vi "ER2007 Calibration Panel.vi"() -> ()   [LabVIEW 2013]
doc: "This vi is used to display and assign calibration parameters to A/D, D/A, and digital I/O channels. These parameters are grouped by channel type (i.e., A/D, D/A, etc) and displayed on separate pages. The user selects a page for review and/or modification using the text ring at the top of the page; changes to a page are saved by pressing the \"Save Page\" button. The calibration coefficients are used to convert voltages to engineering values and vice versa. When a channel is re-calibrated, the new coefficients should be entered here. To permanently store changes, you must press \"Save Page\" for the appropriate channel first. This enables the \"OK\" button at the bottom right of the screen; press this button to save the new value(s) to the calibration file. (The calibration file is read at startup inside the Main Panel vi.) Press \"Cancel\" to restore previous values. AutoCon, Inc., 6/98"
uses:
  Controls/Global ER2007.vi
panel:
  in  "Set":bool
  out "VersionLabel":string="Program JackScrew, Version 0.01, Rolls Royce Gear Systems, Copyright 2000, All Rights Reserved"
  in  "OK":bool
  in  "Cancel":bool
  in  "SavePage":bool
  in  "HW Configuration":u16[](array[ring]) items=["Not Configured", "Bipolar, -10V to +10V", "Unipolar, 0 to +10V", "Bipolar, -5V to +5V", "Unipolar, 0 to +5V", "<reserved>", "<reserved>", "<reserved>", "<reserved>", "<reserved>", "<reserved>", "Digital Input", "Digital Output", "Counter Input"]
  in  "Factor":sgl[](array[numeric]) format="%.5f"
  in  "Zeroes":sgl[](array[numeric]) format="%.5f"
  in  "Page #":u16(ring) items=["Dev 1 PCI-6220 Port 0 DigOut Chls 0-7 DOUT", "Dev 1 PCI-6220 Port 1 DigOut Chls 0-7 DOUT", "Dev 1 PCI-6220 Port 2 DigIn Chls 0-7 DIN", "Dev 1 PCI-6220 Analog In Chls 0-15 AIN", "Dev 2 PCI-6224 Port 0 DigOut Chls 0-7 DOUT", "Dev 2 PCI-6224 Port 0 DigOut Chls 8-15 DOUT", "Dev 2 PCI-6224 Port 1 DigOut Chls 0-7 DOUT", "Dev 2 PCI-6224 Port 2 DigIn Chls 0-7 DIN", "Dev 2 PCI-6224 Analog In Chls 0-15 AIN", "Dev 2 PCI-6224 Analog In Chls 16-31 AIN", "Net 0 Galil CDS 3310", "GPIB 0 IEEE-488 Interface Addr"]
  out "Chl #":string[](array[string])
  in  "Channel Description":string[](array[string])
  in  "Units":string[](array[string])
  # "Calibration Panel"
  # "Note: Units of \"psia\", \"Volts\" and\n\"deg-C\" have special zero routines"
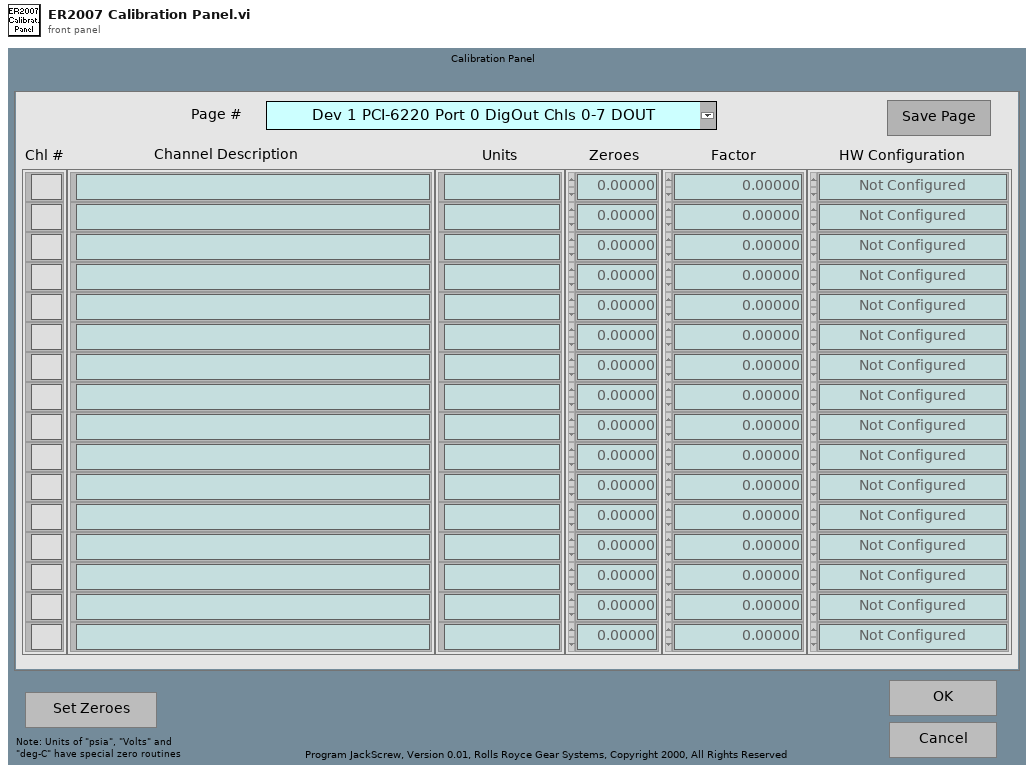
[diagram p1: front panel]
types:
  T1 = cluster{"PageTitle":string, "NumLines":i32, "ChlNum":string[], "ChlDesc":string[], "ChlUnits":string[], "ChlZero":sgl[], "ChlFactor":sgl[], "ChlConfig":u16[]}[]
  T2 = cluster{"PageTitle":string, "NumLines":i32, "ChlNum":string[], "ChlDesc":string[], "ChlUnits":string[], "ChlZero":sgl[], "ChlFactor":sgl[], "ChlConfig":u16[]}
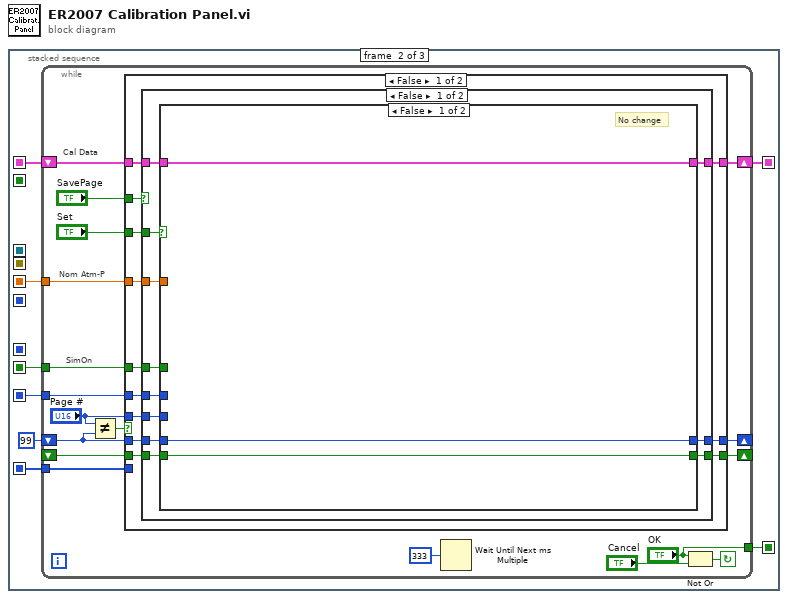
[diagram p0: block diagram]
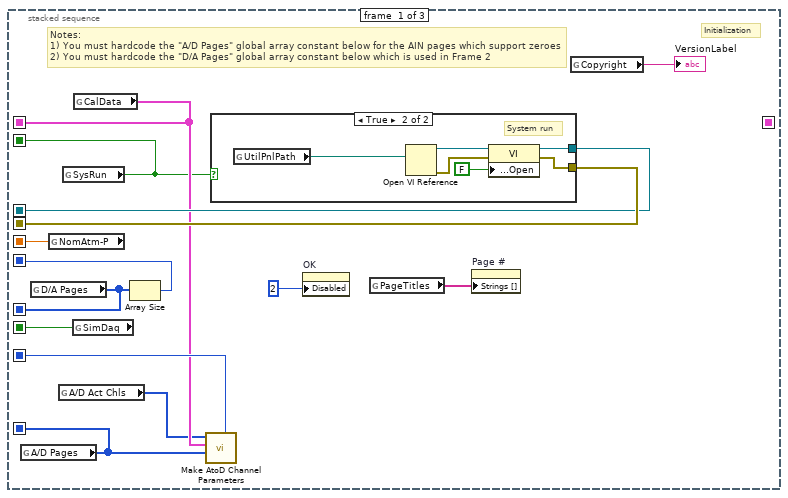
[diagram p2: hidden frame]
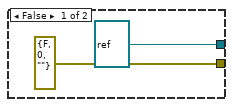
[diagram p3: hidden frame]
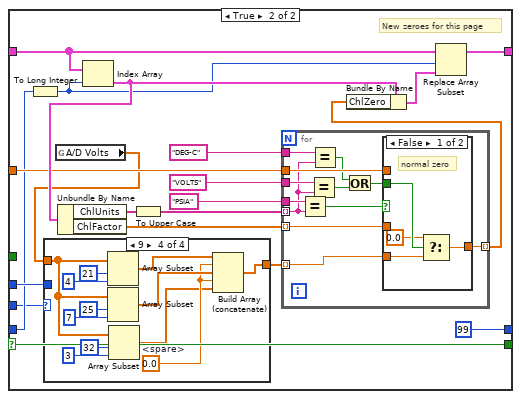
[diagram p5: hidden frame]
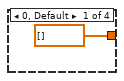
[diagram p6: hidden frame]
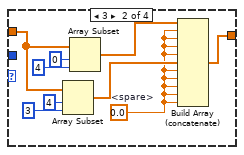
[diagram p7: hidden frame]
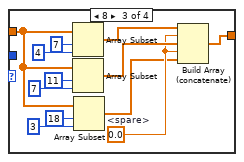
[diagram p8: hidden frame]
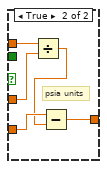
[diagram p9: hidden frame]
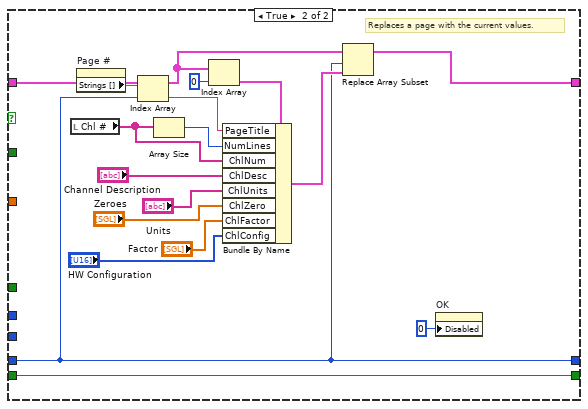
[diagram p10: hidden frame]
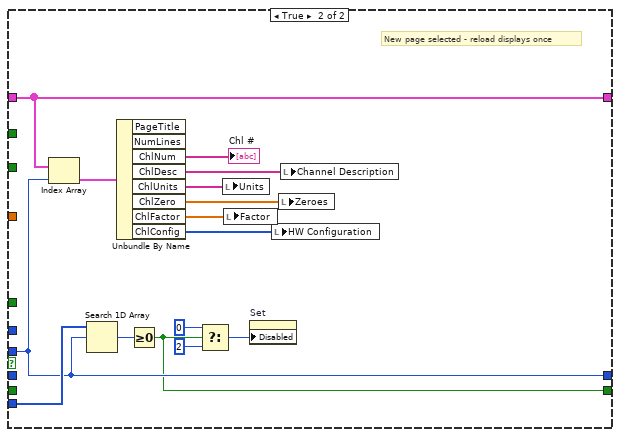
[diagram p11: hidden frame]
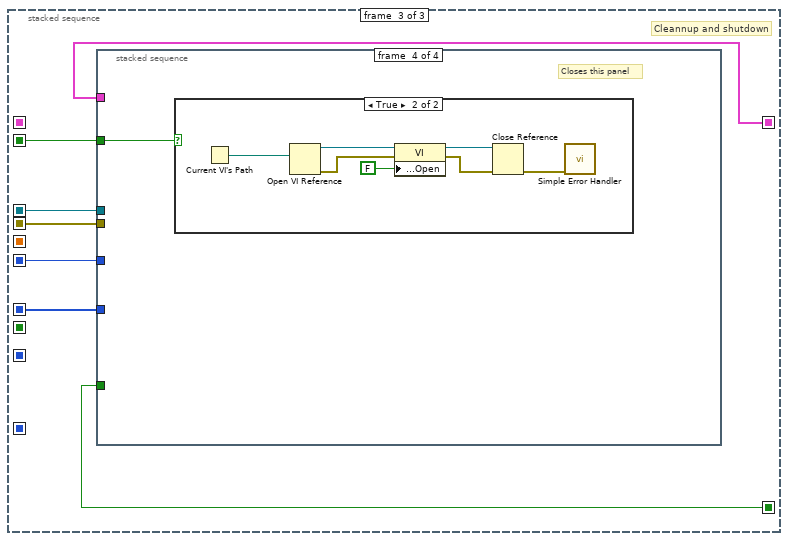
[diagram p12: hidden frame]
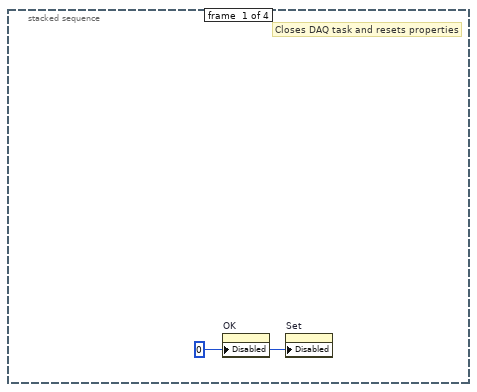
[diagram p13: hidden frame]
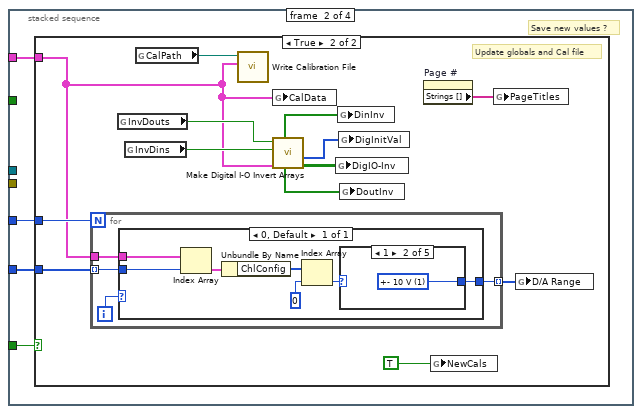
[diagram p14: hidden frame]
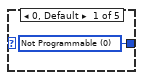
[diagram p16: hidden frame]
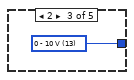
[diagram p17: hidden frame]
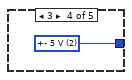
[diagram p18: hidden frame]
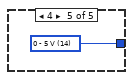
[diagram p19: hidden frame]
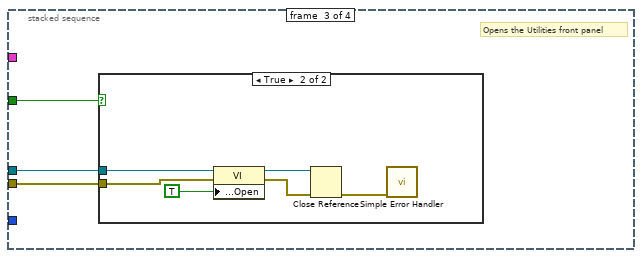
[diagram p20: hidden frame]
diagram:
  n1 = stacked-sequence {
    seq-local: [_ w28 _] -> [_ _ w201]
    seq-local: [w8 _ _] -> [_ w30 _]
    seq-local: [_ w27 _] -> [_ _ w200]
    seq-local: [w4 _ _] -> [_ w26 _]
    seq-local: [w6 _ _] -> [_ w25 _]
    seq-local: [w2 _ _] -> [_ w24 _]
    seq-local: [w13 _ _] -> [_ _ w199]
    seq-local: [w5 _ _] -> [_ _ w198]
    seq-local: [w12 _ _] -> [_ w23 _]
    seq-local: [w7 _ _] -> [_ _ w197]
    seq-local: [w10 _ _] -> [_ _ w196]
    seq-local: [w11 _ _] -> [_ _ w195]
    frame #0 {
      # "Notes:\n1) You must hardcode the \"A/D Pages\" global array constant below for the AIN pages which support zeroes\n2) You must hardcode the \"D/A Pages\" global array constant below which is used in Frame 2"
      # "Initialization"
      n2 = global read "Global ER2007.vi" "A/D Pages"() -> (w2:i32[])
      n3 = global read "Global ER2007.vi" "D/A Pages"() -> (w5:i32[])
      n4 = global read "Global ER2007.vi" "NomAtm-P"() -> (w6:dbl)
      n5 = global read "Global ER2007.vi" "A/D Act Chls"() -> (w3:i32[])
      n6 = global read "Global ER2007.vi" "SysRun"() -> (w7:bool)
      n7 = global read "Global ER2007.vi" "SimDaq"() -> (w4:bool)
      n8 = global read "Global ER2007.vi" "CalData"() -> (w8:T1)
      n9 = Array Size(array=w5) -> (size(s)=w13:i32)
      n10 = call "Make AtoD Channel Parameters.vi"("A/D Pages"=w2, "CalData"=w8, "A/D Active Chl List"=w3) -> ("NumChls"=w12:i32)  [unwired: 2 in, 6 out]
      n11 = case shown="True" w7 {
        tunnel: [refnum<vi> refnum w19] -> w10
        tunnel: [errorcluster {"status"=FALSE, "code"=0, "source"=""} ("error out") w18] -> w11
        frame False {
        }
        frame True {
          # "System run"
          n12 = global read "Global ER2007.vi" "UtilPnlPath"() -> (w17:path)
          n13 = Open VI Reference(vi path=w17) -> (vi reference=w22:refnum<vi>, error out=w21:errorcluster)  [unwired: 5 in]
          n14 = property class="VI"(reference=w22, error in=w21, "Front Panel Window:Open"=FALSE) -> (reference out=w19:refnum<vi>, error out=w18:errorcluster)
        }
      }
      n15 = property on="OK" class="Bool"("Disabled"=u8 2) -> ()  [unwired: 2 in, 2 out]
      n16 = global read "Global ER2007.vi" "PageTitles"() -> (w1:string[])
      n17 = property on="Page #" class="Ring (strict)"("Strings []"=w1) -> ()  [unwired: 2 in, 2 out]
      n18 = global read "Global ER2007.vi" "Copyright"() -> (→"VersionLabel":string)
    }
    frame #1 {
      n19 = while {
        tunnel: w25 -> [w35]
        tunnel: w26 -> [w36]
        tunnel: ["OK"] -> w28
        shift-left: u16 99 -> [w46]
        shift-right: [w44] -> _
        shift-left: w30 -> [w47]
        shift-right: [w43] -> w27
        tunnel: w24 -> [w34]
        tunnel: w23 -> [w33]
        shift-right: [w32] -> _
        shift-left: _ -> [w31]
        stop <- w40 continue-if-true
        # "Cal Data"
        # "SimOn"
        # "Nom Atm-P"
        n20 = Not Equal?(x="Page #", y=w46) -> (x != y?=w48:bool)
        n21 = case shown="False" w48 {
          tunnel: w47 -> [w60 w194]
          tunnel: w46 -> [w57 _]
          tunnel: "Page #" -> [w49 w183]
          tunnel: [w56 w183] -> w44
          tunnel: [w59 w194] -> w43
          tunnel: "SavePage" -> [w58 _]
          tunnel: "Set" -> [w55 _]
          tunnel: w36 -> [w54 _]
          tunnel: w35 -> [w53 _]
          tunnel: w34 -> [_ w184]
          tunnel: w33 -> [w52 _]
          tunnel: [w50 w181] -> w32
          tunnel: w31 -> [w51 _]
          frame False {
            n22 = case shown="False" w58 {
              tunnel: w60 -> [w70 w171]
              tunnel: [w71 w169] -> w59
              tunnel: w57 -> [w67 w165]
              tunnel: [w68 w165] -> w56
              tunnel: w55 -> [w69 _]
              tunnel: w54 -> [w66 _]
              tunnel: w53 -> [w65 _]
              tunnel: w52 -> [w64 _]
              tunnel: w51 -> [w63 w164]
              tunnel: [w62 w164] -> w50
              tunnel: w49 -> [w61 _]
              frame False {
                n23 = case shown="False" w69 {
                  tunnel: [w74 w83] -> w71
                  tunnel: w70 -> [w74 w82]
                  tunnel: [w73 w84] -> w68
                  tunnel: w67 -> [w73 w77]
                  tunnel: w66 -> [_ w81]
                  tunnel: w65 -> [_ w80]
                  tunnel: w64 -> [_ w79]
                  tunnel: w63 -> [w72 w78]
                  tunnel: [w72 w76] -> w62
                  tunnel: w61 -> [_ w75]
                  frame False {
                    # "No change"
                  }
                  frame True {
                    n24 = case shown="False" w78 {
                      selector: w78 -> [w86 w92]
                      tunnel: [w85 u16 99] -> w84
                      tunnel: [w87 w104] -> w83
                      tunnel: w82 -> [w87 w103]
                      tunnel: w81 -> [_ _]
                      tunnel: w80 -> [_ w96]
                      tunnel: w79 -> [_ w93]
                      tunnel: w77 -> [w85 w90]
                      tunnel: [w86 w92] -> w76
                      tunnel: w75 -> [_ w89]
                      frame False {
                        # "This page does not support zeroing"
                      }
                      frame True {
                        # "New zeroes for this page"
                        n25 = To Long Integer(number=w90) -> (32bit integer=w100:i32)
                        n26 = global read "Global ER2007.vi" "A/D Volts"() -> (w88:dbl[])
                        n27 = case shown="9" w89 {
                          tunnel: [dbl[] [] w114 w118 w130] -> w95
                          tunnel: w93 -> [_ _ _ _]
                          tunnel: w88 -> [_ w111 w120 w132]
                          frame 0, Default {
                          }
                          frame 3 {
                            w109 = 0.0  # <spare>
                            n28 = Array Subset(array=w111, index=4, length=3) -> (w110:dbl[])
                            n29 = Array Subset(array=w111, index=0, length=4) -> (w115:dbl[])
                            n30 = Build Array (concatenate)(w115, w109, w109, w109, w109, w110, w109, w109, w109, w109, w109) -> (w114:dbl[])
                          }
                          frame 8 {
                            w121 = 0.0  # <spare>
                            n31 = Array Subset(array=w120, index=7, length=4) -> (w127:dbl[])
                            n32 = Array Subset(array=w120, index=11, length=7) -> (w124:dbl[])
                            n33 = Array Subset(array=w120, index=18, length=3) -> (w119:dbl[])
                            n34 = Build Array (concatenate)(w127, w121, w124, w121, w119) -> (w118:dbl[])
                          }
                          frame 9 {
                            w133 = 0.0  # <spare>
                            n35 = Array Subset(array=w132, index=21, length=4) -> (w139:dbl[])
                            n36 = Array Subset(array=w132, index=25, length=7) -> (w136:dbl[])
                            n37 = Array Subset(array=w132, index=32, length=3) -> (w131:dbl[])
                            n38 = Build Array (concatenate)(w139, w133, w136, w133, w131) -> (w130:dbl[])
                          }
                        }
                        n39 = Index Array(array=w103, index=w100) -> (element=w102:T2)
                        n40 = Unbundle By Name(w102) -> ("ChlUnits"=w107:string[], "ChlFactor"=w99:sgl[])
                        n41 = To Upper Case(1:w107) -> (0:w106:string[])
                        n42 = for {
                          tunnel: w95 -> [w142] mode=indexing
                          tunnel: w106 -> [w147] mode=indexing
                          tunnel: "PSIA" -> [w153]
                          tunnel: [w151] -> w98 mode=indexing
                          tunnel: w99 -> [w150] mode=indexing
                          tunnel: w96 -> [w149]
                          tunnel: "VOLTS" -> [w148]
                          tunnel: "DEG-C" -> [w146]
                          n43 = Equal?(x=w153, y=w147) -> (x = y?=w152:bool)
                          n44 = Equal?(x=w148, y=w147) -> (x = y?=w144:bool)
                          n45 = Equal?(x=w146, y=w147) -> (x = y?=w143:bool)
                          n46 = Or(x=w143, y=w144) -> (x .or. y?=w145:bool)
                          n47 = case shown="False" w152 {
                            tunnel: [w154 w159] -> w151
                            tunnel: w142 -> [w156 w160]
                            tunnel: w150 -> [_ w161]
                            tunnel: w149 -> [_ w162]
                            tunnel: w145 -> [w157 _]
                            frame False {
                              # "normal zero"
                              n48 = Select(t=0.0, s=w157, f=w156) -> (s? t:f=w154:dbl)
                            }
                            frame True {
                              # "psia units"
                              n49 = Divide(x=w162, y=w161) -> (x/y=w158:dbl)
                              n50 = Subtract(x=w160, y=w158) -> (x-y=w159:dbl)
                            }
                          }
                        }
                        n51 = Bundle By Name(cluster=w102, "ChlZero"=w98) -> (w101:T2)
                        n52 = Replace Array Subset(array=w103, new element=w101, index=w100) -> (w104:T1)
                      }
                    }
                  }
                }
              }
              frame True {
                # "Replaces a page with the current values."
                n53 = local read "Chl #"() -> (w163:string[])
                n54 = property on="Page #" class="Ring (strict)"() -> ("Strings []"=w168:string[])  [unwired: 2 in, 2 out]
                n55 = Index Array(array=w168, index=w165) -> (element=w167:string)
                n56 = Array Size(array=w163) -> (size(s)=w172:i32)
                n57 = Index Array(array=w171, index=0 ("Index")) -> (element=w178:T2)
                n58 = Bundle By Name(cluster=w178, "PageTitle"=w167, "NumLines"=w172, "ChlNum"=w163, "ChlDesc"="Channel Description", "ChlUnits"="Units", "ChlZero"="Zeroes", "ChlFactor"="Factor", "ChlConfig"="HW Configuration") -> (w170:T2)
                n59 = Replace Array Subset(array=w171, new element=w170, index=w165) -> (w169:T1)
                n60 = property on="OK" class="Bool"("Disabled"=u8 0) -> ()  [unwired: 2 in, 2 out]
              }
            }
          }
          frame True {
            # "New page selected - reload displays once"
            n61 = Index Array(array=w194, index=w183) -> (element=w193:T2)
            n62 = Search 1D Array(1D array=w184, element=w183) -> (index of element=w182:i32)  [unwired: 1 in]
            n63 = Unbundle By Name(w193) -> ("ChlNum"=→"Chl #":string[], "ChlDesc"=w188:string[], "ChlUnits"=w189:string[], "ChlZero"=w190:sgl[], "ChlFactor"=w191:sgl[], "ChlConfig"=w192:u16[])  [unwired: 2 out]
            n64 = Greater Or Equal To 0?(x=w182) -> (x >= 0?=w181:bool)
            n65 = Select(t=u8 0 ("Disabled"), s=w181, f=u8 2) -> (s? t:f=w186:u8)
            n66 = local write "Units"(w189) -> ()
            n67 = local write "Factor"(w191) -> ()
            n68 = property on="Set" class="Bool"("Disabled"=w186) -> ()  [unwired: 2 in, 2 out]
            n69 = local write "HW Configuration"(w192) -> ()
            n70 = local write "Zeroes"(w190) -> ()
            n71 = local write "Channel Description"(w188) -> ()
          }
        }
        n72 = Wait Until Next ms Multiple(millisecond multiple=u32 333) -> ()  [unwired: 1 out]
        n73 = Not Or(1:"Cancel", 2:"OK") -> (0:w40:bool)
      }
    }
    frame #2 {
      # "Cleannup and shutdown"
      n74 = stacked-sequence {
        tunnel: w201 -> [_ w206 _ _]
        tunnel: w200 -> [_ w205 _ _]
        tunnel: w199 -> [_ w204 _ _]
        tunnel: w198 -> [_ w203 _ _]
        tunnel: w197 -> [_ _ w238 w245]
        tunnel: w196 -> [_ _ w237 _]
        tunnel: w195 -> [_ _ w236 _]
        frame #0 {
          w202 = u8 0 ("Write Attribute")
          # "Closes DAQ task and resets properties"
          n75 = property on="OK" class="Bool"("Disabled"=w202) -> ()  [unwired: 2 in, 2 out]
          n76 = property on="Set" class="Bool"("Disabled"=w202) -> ()  [unwired: 2 in, 2 out]
        }
        frame #1 {
          # "Save new values ?"
          n77 = case shown="True" w206 {
            tunnel: w205 -> [_ w208]
            tunnel: w204 -> [_ w219]
            tunnel: w203 -> [_ w218]
            frame False {
            }
            frame True {
              # "Update globals and Cal file"
              n78 = for {
                N: w219 -> [_]
                tunnel: w208 -> [w222]
                tunnel: [w221] -> w209 mode=indexing
                tunnel: w218 -> [w220] mode=indexing
                i -> [w223]
                n79 = case shown="0, Default" w223 {
                  tunnel: w222 -> [w225]
                  tunnel: [w226] -> w221
                  tunnel: w220 -> [w224]
                  frame 0, Default {
                    n80 = Index Array(array=w225, index=w224) -> (element=w230:T2)
                    n81 = Unbundle By Name(w230) -> ("ChlConfig"=w229:u16[])
                    n82 = Index Array(array=w229, index=0 ("Index")) -> (element=w227:u16)
                    n83 = case shown="1" w227 {
                      tunnel: [w231 w232 w233 w234 w235] -> w226
                      frame 0, Default {
                        w231 = 0 items=["Not Programmable", "+- 10 V", "+- 5 V", "+- 2.5 V", "+- 1.67 V", "+- 1.25 V", "+- 1 V", "+- .625 V", "+- .5 V", "+- .1 V", "+- .05 V", "+- .01 V", "+- .005 V", "0 - 10 V", "0 - 5 V", "0 - 2.5 V", "0 - 2 V", "0 - 1.67 V", "0 - 1.25 V", "0 - 1 V", "0 - .1 V", "0 - .01 V", "4-20 mA", "2-10 mA", "1-5 mA", "0.5-2.5 mA"] ("DA0Range")
                      }
                      frame 1 {
                        w232 = 1 items=["Not Programmable", "+- 10 V", "+- 5 V", "+- 2.5 V", "+- 1.67 V", "+- 1.25 V", "+- 1 V", "+- .625 V", "+- .5 V", "+- .1 V", "+- .05 V", "+- .01 V", "+- .005 V", "0 - 10 V", "0 - 5 V", "0 - 2.5 V", "0 - 2 V", "0 - 1.67 V", "0 - 1.25 V", "0 - 1 V", "0 - .1 V", "0 - .01 V", "4-20 mA", "2-10 mA", "1-5 mA", "0.5-2.5 mA"] ("DA0Range")
                      }
                      frame 2 {
                        w233 = 13 items=["Not Programmable", "+- 10 V", "+- 5 V", "+- 2.5 V", "+- 1.67 V", "+- 1.25 V", "+- 1 V", "+- .625 V", "+- .5 V", "+- .1 V", "+- .05 V", "+- .01 V", "+- .005 V", "0 - 10 V", "0 - 5 V", "0 - 2.5 V", "0 - 2 V", "0 - 1.67 V", "0 - 1.25 V", "0 - 1 V", "0 - .1 V", "0 - .01 V", "4-20 mA", "2-10 mA", "1-5 mA", "0.5-2.5 mA"] ("DA0Range")
                      }
                      frame 3 {
                        w234 = 2 items=["Not Programmable", "+- 10 V", "+- 5 V", "+- 2.5 V", "+- 1.67 V", "+- 1.25 V", "+- 1 V", "+- .625 V", "+- .5 V", "+- .1 V", "+- .05 V", "+- .01 V", "+- .005 V", "0 - 10 V", "0 - 5 V", "0 - 2.5 V", "0 - 2 V", "0 - 1.67 V", "0 - 1.25 V", "0 - 1 V", "0 - .1 V", "0 - .01 V", "4-20 mA", "2-10 mA", "1-5 mA", "0.5-2.5 mA"] ("DA0Range")
                      }
                      frame 4 {
                        w235 = 14 items=["Not Programmable", "+- 10 V", "+- 5 V", "+- 2.5 V", "+- 1.67 V", "+- 1.25 V", "+- 1 V", "+- .625 V", "+- .5 V", "+- .1 V", "+- .05 V", "+- .01 V", "+- .005 V", "0 - 10 V", "0 - 5 V", "0 - 2.5 V", "0 - 2 V", "0 - 1.67 V", "0 - 1.25 V", "0 - 1 V", "0 - .1 V", "0 - .01 V", "4-20 mA", "2-10 mA", "1-5 mA", "0.5-2.5 mA"] ("DA0Range")
                      }
                    }
                  }
                }
              }
              n84 = global read "Global ER2007.vi" "InvDouts"() -> (w216:bool)
              n85 = global read "Global ER2007.vi" "InvDins"() -> (w215:bool)
              n86 = global read "Global ER2007.vi" "CalPath"() -> (w217:path)
              n87 = call "Write Calibration File.vi"("CalDataIn"=w208, "CalFilepath"=w217) -> ()  [unwired: 6 in]
              n88 = global write "Global ER2007.vi" "CalData"(w208) -> ()
              n89 = call "Make Digital I-O Invert Arrays.vi"("CalDataIn"=w208, "InvDins"=w215, "InvDouts"=w216) -> ("DIO-Inv"=w212:bool[][], "DoutInit"=w211:i32[], "DoutInv (1D)"=w213:bool[], "DinInv (1D)"=w214:bool[])  [unwired: 1 in, 4 out]
              n90 = global write "Global ER2007.vi" "DigIO-Inv"(w212) -> ()
              n91 = global write "Global ER2007.vi" "DinInv"(w214) -> ()
              n92 = global write "Global ER2007.vi" "DigInitVal"(w211) -> ()
              n93 = global write "Global ER2007.vi" "DoutInv"(w213) -> ()
              n94 = property on="Page #" class="Ring (strict)"() -> ("Strings []"=w210:string[])  [unwired: 2 in, 2 out]
              n95 = global write "Global ER2007.vi" "NewCals"(TRUE ("NewCals")) -> ()
              n96 = global write "Global ER2007.vi" "PageTitles"(w210) -> ()
              n97 = global write "Global ER2007.vi" "D/A Range"(w209) -> ()
            }
          }
        }
        frame #2 {
          # "Opens the Utilities front panel"
          n98 = case shown="True" w238 {
            tunnel: w237 -> [_ w244]
            tunnel: w236 -> [_ w243]
            frame False {
              # "Not a System run"
            }
            frame True {
              n99 = property class="VI"(reference=w244, error in=w243, "Front Panel Window:Open"=TRUE) -> (reference out=w241:refnum<vi>, error out=w240:errorcluster)
              n100 = Close Reference(reference=w241, error in (no error)=w240) -> (error out=w239:errorcluster)
              n101 = call <vilib>:"Simple Error Handler.vi"("error in (no error)"=w239) -> ()  [unwired: 4 in, 5 out]
            }
          }
        }
        frame #3 {
          # "Closes this panel"
          n102 = case shown="True" w245 {
            frame False {
            }
            frame True {
              n103 = Current VI's Path() -> (path=w252:path)
              n104 = Open VI Reference(vi path=w252) -> (vi reference=w251:refnum<vi>, error out=w250:errorcluster)  [unwired: 5 in]
              n105 = property class="VI"(reference=w251, error in=w250, "Front Panel Window:Open"=FALSE) -> (reference out=w248:refnum<vi>, error out=w247:errorcluster)
              n106 = Close Reference(reference=w248, error in (no error)=w247) -> (error out=w246:errorcluster)
              n107 = call <vilib>:"Simple Error Handler.vi"("error in (no error)"=w246) -> ()  [unwired: 4 in, 5 out]
            }
          }
        }
      }
    }
  }
